vi "RandomPointGenerator.vi"(6 "Região do campo\nTeste Passe":enum16{"3", "2", "1", "0", "-1", "-2", "-3"}(ring), 9 "Field defense":dbl[](array[numeric]), 10 "IA State Input":T1) -> (2 "Point Ally Field":dbl[](array[numeric]))   [LabVIEW 2017]
uses:
  Core/AI Input.ctl
  Core/AI Robot.ctl
  Intel/Functions Enum.ctl
  Intel/AttackerStates.ctl
  Path Planning/RRT/PathDests.ctl
  Path Planning/RRT/PathDest.ctl
  Core/AI Ball.ctl
  Core/Field Size.ctl
  Core/AI Judge.ctl
  Intel/Command Enum.ctl
  Util/Events/Events.ctl
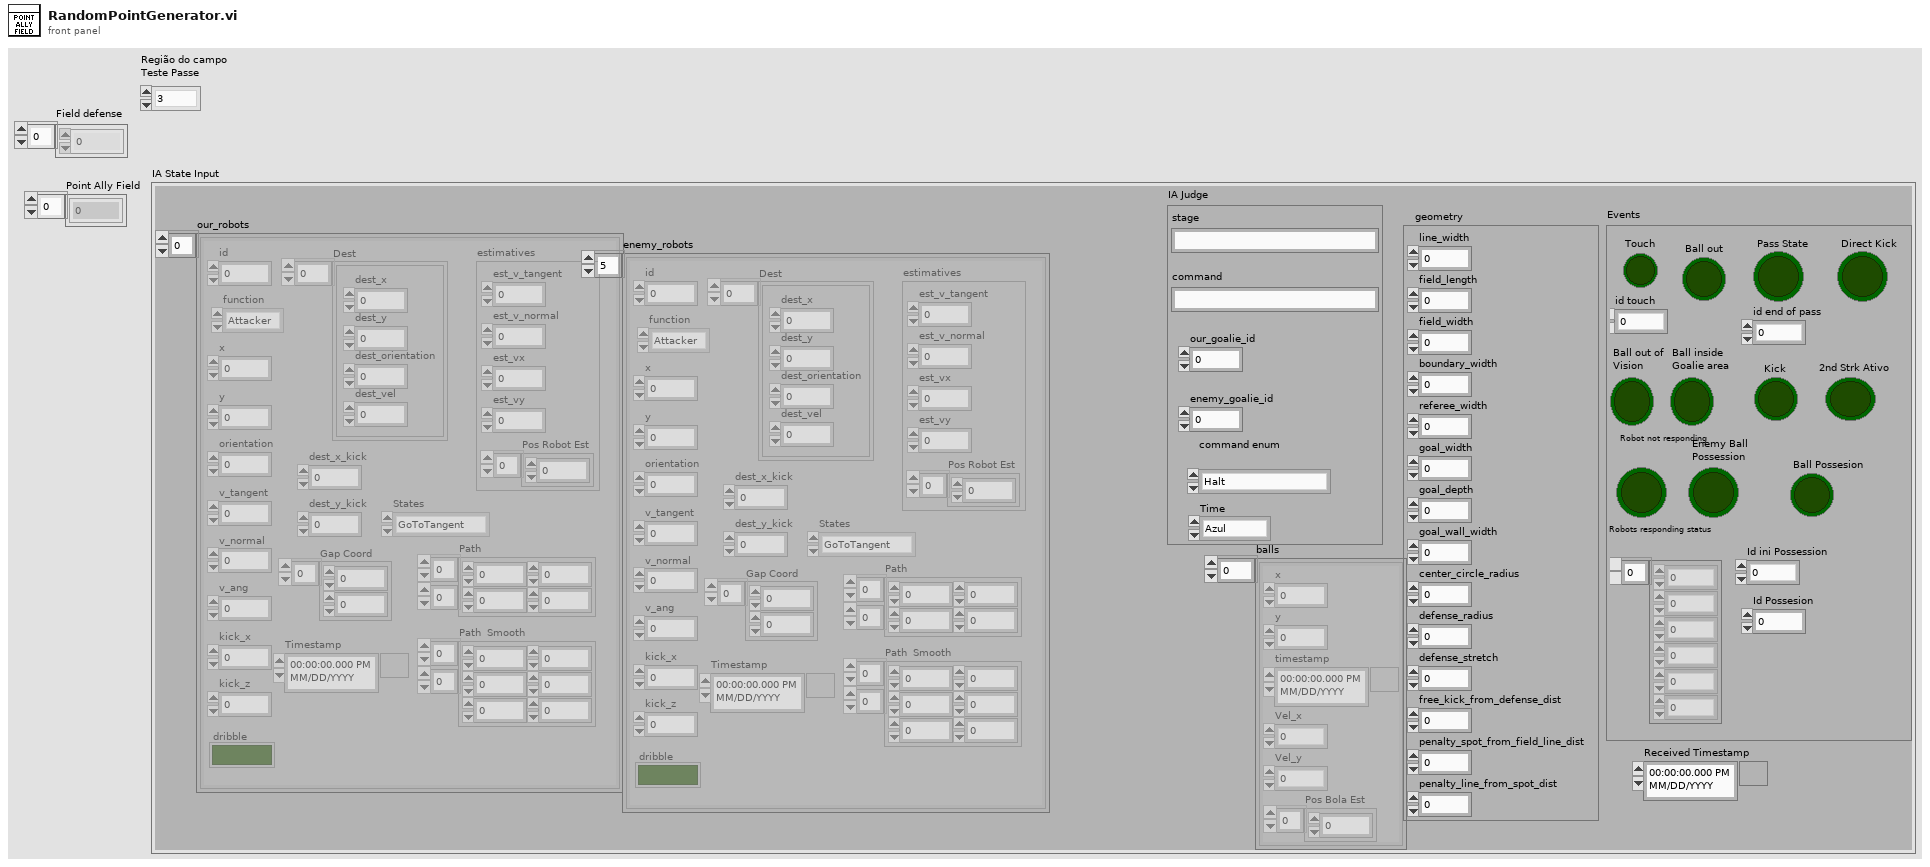
[diagram p1: front panel]
types:
  T1 = typedef "AI Input.ctl" = cluster{"our_robots":T2[], "enemy_robots":T2[], "balls":T7[], "geometry":T8, "IA Judge":T9, "Received Timestamp":timestamp, "Events":T11}
  T2 = typedef "AI Robot.ctl" = cluster{"id":u32, "function":T3, "x":dbl, "y":dbl, "orientation":dbl, "v_tangent":dbl, "v_normal":dbl, "v_ang":dbl, "kick_x":dbl, "kick_z":dbl, "dribble":bool, "Timestamp":timestamp, "estimatives":cluster{"est_v_tangent":dbl, "est_v_normal":dbl, "est_vx":dbl, "est_vy":dbl, "Pos Robot Est":dbl[]}, "dest_x_kick":dbl, "dest_y_kick":dbl, "Gap Coord":dbl[], "States":T4, "Path ":dbl[][], "Path  Smooth":dbl[][], "Dest":T5}
  T3 = typedef "Functions Enum.ctl" = enum16{"2nd Striker", "Attacker", "Goalie", "Defender", "Striker", "Goto 0", "Dummy", "Kicker", "ZigZag 0", "ZigZag 1", "ZigZag 2", "ZigZag 3", "ZigZag 4", "ZigZag 5", "ZigZag 6", "ZigZag 7", "ZigZag 8", ""}
  T4 = typedef "AttackerStates.ctl" = enum16{"Pass", "GoToTangent", "BallGetting", "GoToKick", ""}
  T5 = typedef "PathDests.ctl" = T6[]
  T6 = typedef "PathDest.ctl" = cluster{"dest_x":dbl, "dest_y":dbl, "dest_orientation":dbl, "dest_vel":dbl}
  T7 = typedef "AI Ball.ctl" = cluster{"x":dbl, "y":dbl, "timestamp":timestamp, "Vel_x":dbl, "Vel_y":dbl, "Pos Bola Est":dbl[]}
  T8 = typedef "Field Size.ctl" = cluster{"line_width":u32, "field_length":u32, "field_width":u32, "boundary_width":u32, "referee_width":u32, "goal_width":u32, "goal_depth":u32, "goal_wall_width":u32, "center_circle_radius":u32, "defense_radius":u32, "defense_stretch":u32, "free_kick_from_defense_dist":u32, "penalty_spot_from_field_line_dist":u32, "penalty_line_from_spot_dist":u32}
  T9 = typedef "AI Judge.ctl" = cluster{"stage":string, "command":string, "our_goalie_id":dbl, "enemy_goalie_id":dbl, "command enum":T10, "Time":enum16{"Azul", "Amarelo"}}
  T10 = typedef "Command Enum.ctl" = enum16{"Halt", "Stop", "Force Start", "PKA Normal Start", "Prepare Kickoff Ally", "PKE Normal Start", "Prepare Kickoff Enemy", "Prepare Penalty Ally", "PPA Normal Start", "Prepare Penalty Enemy", "PPE Normal Start", "Direct Free Enemy", "Direct Free Ally", "Indirect Free Enemy", "Indirect Free Ally", "Timeout Enemy", "Timeout Ally", "Goal Enemy", "Goal Ally", "Ball Placement Enemy", "Ball Placement Ally", "Normal Half Time", "Extra Time Break", "Extra Half Time", "None", "Post Game"}
  T11 = typedef "Events.ctl" = cluster{"Touch":bool, "Ball out":bool, "id touch":dbl, "Ball out of \nVision":bool, "Ball inside \nGoalie area":bool, "Robot not responding":bool, "Robots responding status":dbl[], "Enemy Ball \nPossession":bool, "Pass State":bool, "id end of pass":dbl, "Kick":bool, "Id ini Possession":dbl, "Ball Possesion":bool, "Id Possesion":dbl, "Direct Kick":bool, "2nd Strk Ativo":bool}
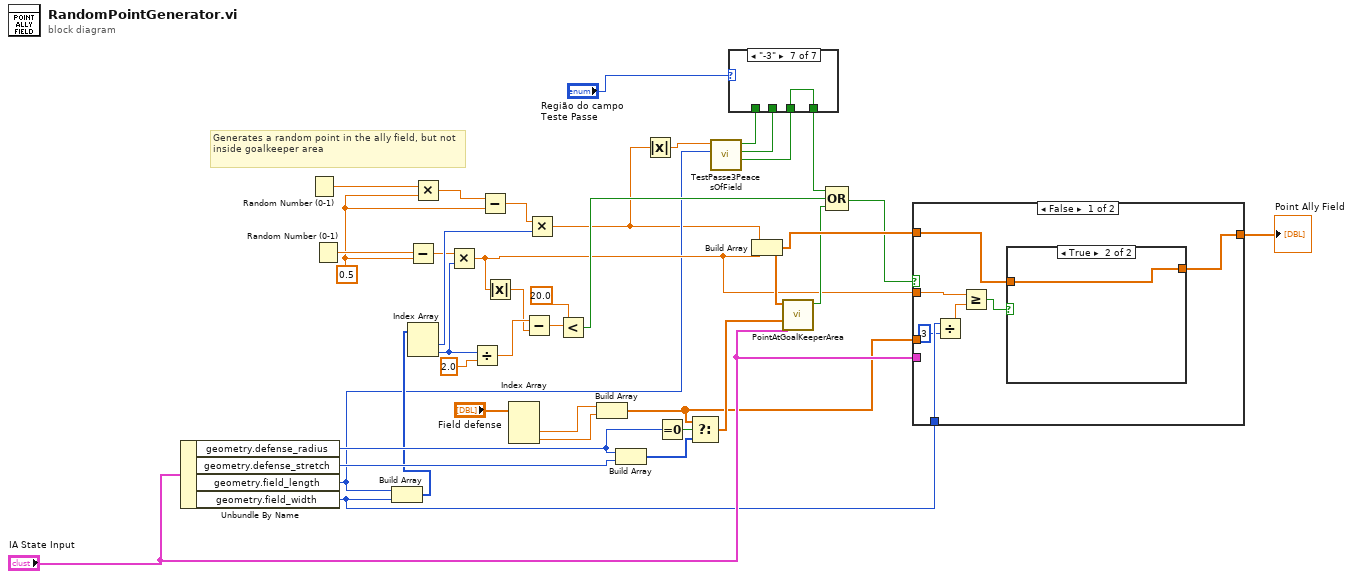
[diagram p0: block diagram]
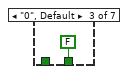
[diagram p4: hidden frame]
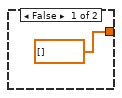
[diagram p8: hidden frame]
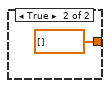
[diagram p9: hidden frame]
diagram:
  w34 = 0.5 ("y")
  # "Generates a random point in the ally field, but not inside goalkeeper area"
  n1 = Unbundle By Name("IA State Input") -> ("geometry.defense_radius"=w18:u32, "geometry.defense_stretch"=w20:u32, "geometry.field_length"=w7:u32, "geometry.field_width"=w9:u32)
  n2 = Random Number (0-1)() -> (number: 0 to 1=w36:dbl)
  n3 = Random Number (0-1)() -> (number: 0 to 1=w37:dbl)
  n4 = Build Array(w7, w9) -> (w15:u32[])
  n5 = Subtract(x=w37, y=w34) -> (x-y=w38:dbl)
  n6 = Index Array(array=w15) -> (element #1=w39:u32, element #2=w30:u32)  [unwired: 2 in]
  n7 = Multiply(x=w36, y=w34) -> (x*y=w35:dbl)
  n8 = Multiply(x=w38, y=w30) -> (x*y=w10:dbl)
  n9 = Divide(x=w30, y=2.0) -> (x/y=w28:dbl)
  n10 = Subtract(x=w35, y=w34) -> (x-y=w33:dbl)
  n11 = Absolute Value(x=w10) -> (abs(x)=w27:dbl)
  n12 = Index Array(array="Field defense") -> (element #2=w13:dbl, element #3=w12:dbl)  [unwired: 3 in, 1 out]
  n13 = Subtract(x=w28, y=w27) -> (x-y=w26:dbl)
  n14 = Multiply(x=w33, y=w39) -> (x*y=w6:dbl)
  n15 = Less?(x=w26, y=20.0) -> (x < y?=w23:bool)
  n16 = Build Array(w13, w12) -> (w11:dbl[])
  n17 = Build Array(w18, w20) -> (w17:u32[])
  n18 = Absolute Value(x=w6) -> (abs(x)=w8:dbl)
  n19 = Equal To 0?(x=w18) -> (x = 0?=w19:bool)
  n20 = Select(t=w11, s=w19, f=w17) -> (s? t:f=w16:dbl[])
  n21 = call "TestPasse3PeacesOfField.vi"("Field Length"=w7, "X"=w8) -> ("Terceiro Terço"=w1:bool, "Segundo Terço"=w2:bool, "Primeiro Terço"=w3:bool)  [unwired: 7 in]
  n22 = case shown="\"-3\"" "Região do campo\nTeste Passe" {
    tunnel: w1 -> [_ _ _ _ _ w45 w46]
    tunnel: [w40 w41 FALSE ("Terceiro Terço") w43 w44 w45 w46] -> w4
    tunnel: w2 -> [w40 _ _ _ w44 _ _]
    tunnel: w3 -> [_ w41 _ w43 _ _ _]
    frame "-2" {
    }
    frame "-1" {
    }
    frame "0", Default {
    }
    frame "1" {
    }
    frame "2" {
    }
    frame "3" {
    }
    frame "-3" {
    }
  }
  n23 = Build Array(w6, w10) -> (w32:dbl[])
  n24 = call "PointAtGoalKeeperArea.vi"("Field defense"=w16, "IA State Input"="IA State Input", "Array"=w32) -> ("Point inside goalkeeper area ?"=w24:bool)  [unwired: 8 in]
  n25 = Compound Arithmetic op=OR(w4, w23, w24) -> (w22:bool)
  n26 = case shown="False" w22 {
    tunnel: [w48 dbl[] []] -> w31
    tunnel: w32 -> [w47 _]
    tunnel: "IA State Input" -> [_ _]
    tunnel: w11 -> [_ _]
    tunnel: w10 -> [w53 _]
    tunnel: w9 -> [w52 _]
    frame False {
      n27 = Divide(x=w52, y=u32 3) -> (x/y=w50:dbl)
      n28 = Greater Or Equal?(x=w53, y=w50) -> (x >= y?=w49:bool)
      n29 = case shown="True" w49 {
        tunnel: [dbl[] [] w55] -> w48
        tunnel: w47 -> [_ w55]
        frame False {
        }
        frame True {
        }
      }
    }
    frame True {
    }
  }
  "Point Ally Field" <- w31
